vi "labview与三菱PLC通讯(main).vi"(0 "读取=0写入=1":i16, 1 "变量类型":u32(ring) items=["X", "Y", "M", "D"], 2 "PLC地址":string, 3 "PLC数据":string, 4 "16位/32位":u32(ring) items=["16bit", "32bit"], 6 "端口选择":refnum<visa-resource-name>, 8 "波特率":u32(ring) items=["9600"=9600, "19200"=19200, "115200"=115200], 10 "校检":u32(ring) items=["无", "偶", "奇"], 12 "数据位":u32(ring) items=["7"=7, "8"=8]) -> (14 "读取数据输出":u32, 15 "读取成功":bool, 17 "写入成功":bool)   [LabVIEW 2015, in "PLC.lvlib"]
uses:
  PLC.lvlib
panel:
  out "写入PLC变量命令":string
  out "十六进制整型字符串 2":string
  out "十六进制整型字符串":string
  out "长度":i32
  out "数据":string
  out "数字 2":u32
  out "地址偏移量":string="240"
  out "读取PLC变量命令":string
  out "读取为0写入为1":string="1"
  out "校验码2":string
  out "校验码1":string
  out "数字":u16
  out "长度（剩余）":i32=2
  out "变量地址":string
  out "读取返回数据":string
  # "X000-X577"
  # "Y000-Y577"
  # "M0000-M7999"
  # "D0000-D7999"
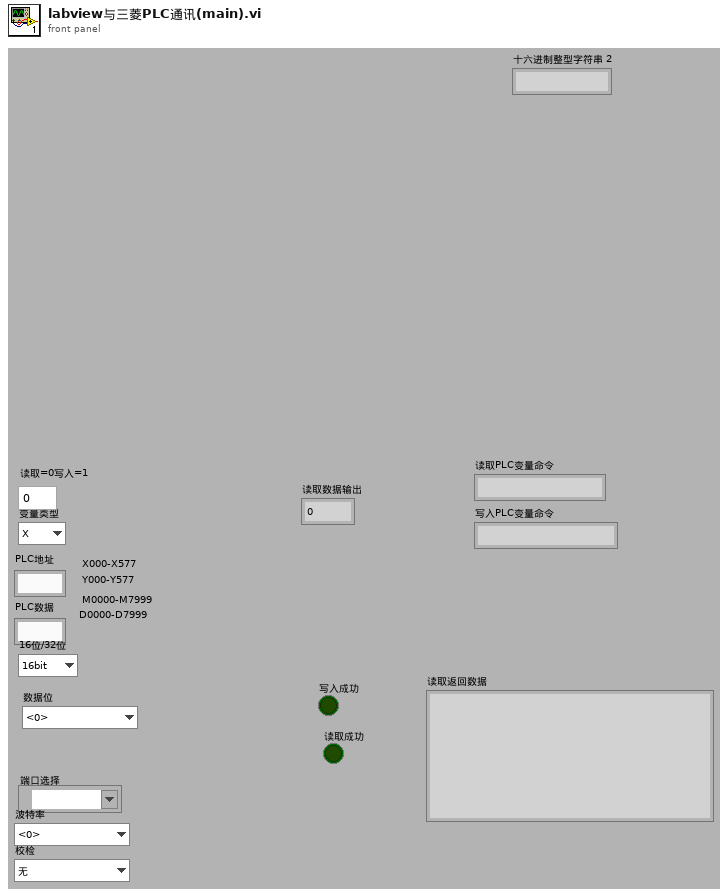
[diagram p1: front panel]
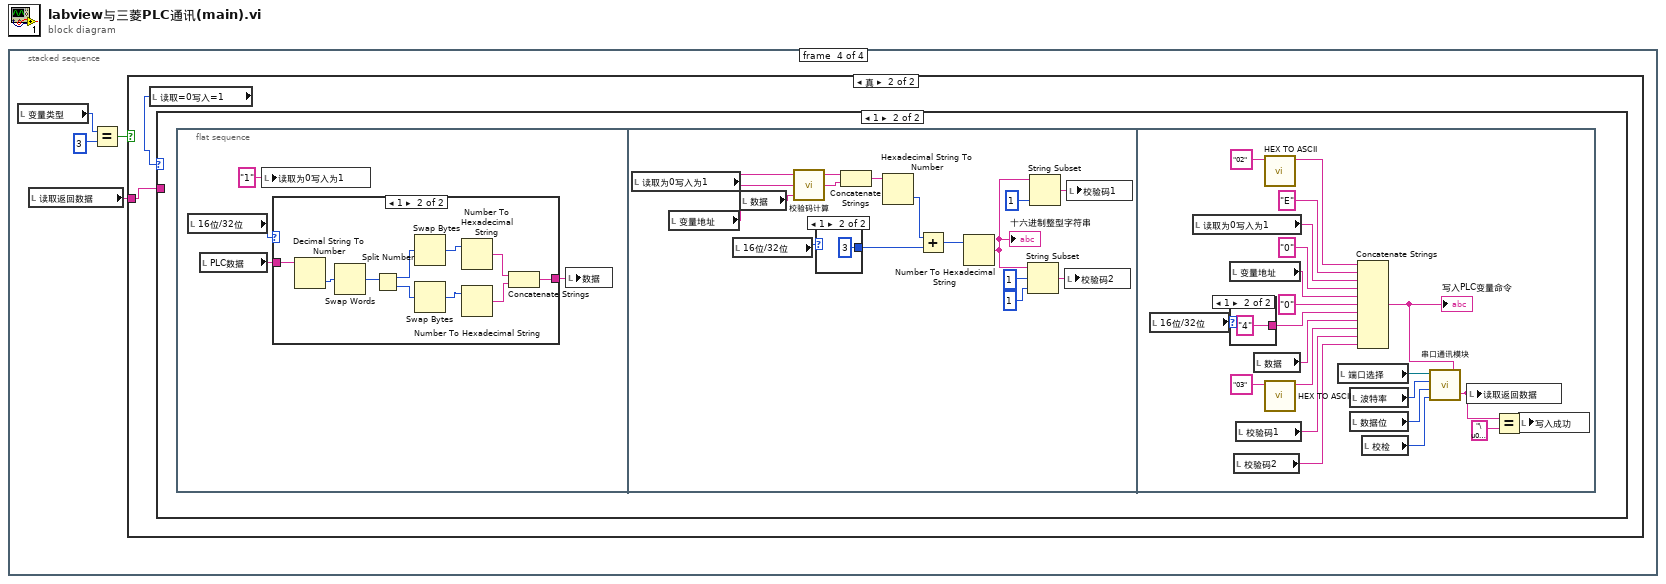
[diagram p0: block diagram]
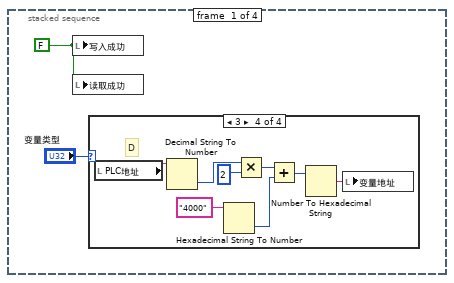
[diagram p2: hidden frame]
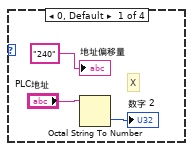
[diagram p3: hidden frame]
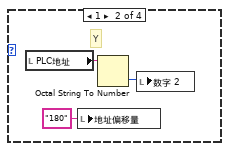
[diagram p4: hidden frame]
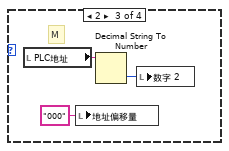
[diagram p5: hidden frame]
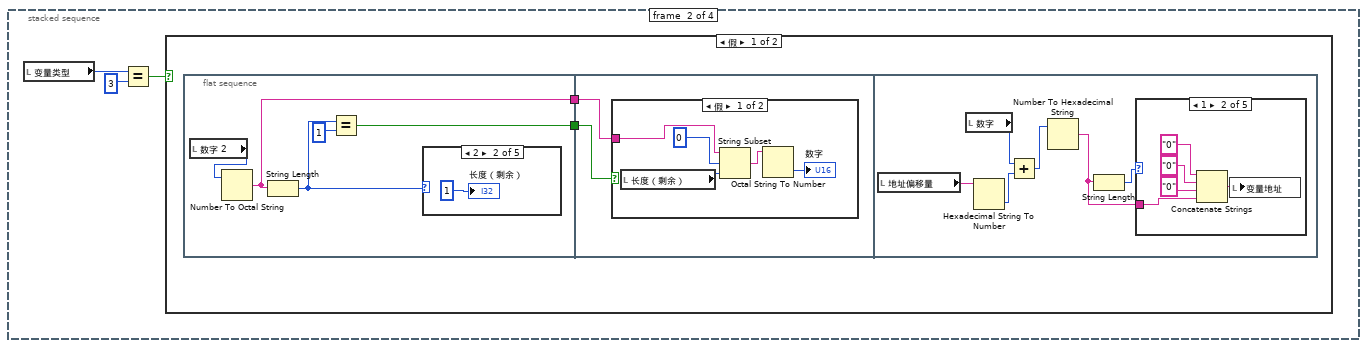
[diagram p6: hidden frame]
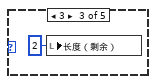
[diagram p8: hidden frame]
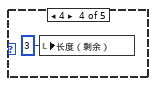
[diagram p9: hidden frame]
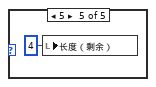
[diagram p10: hidden frame]
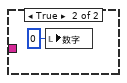
[diagram p11: hidden frame]
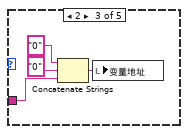
[diagram p13: hidden frame]
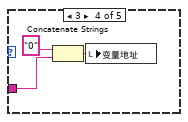
[diagram p14: hidden frame]
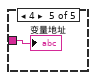
[diagram p15: hidden frame]
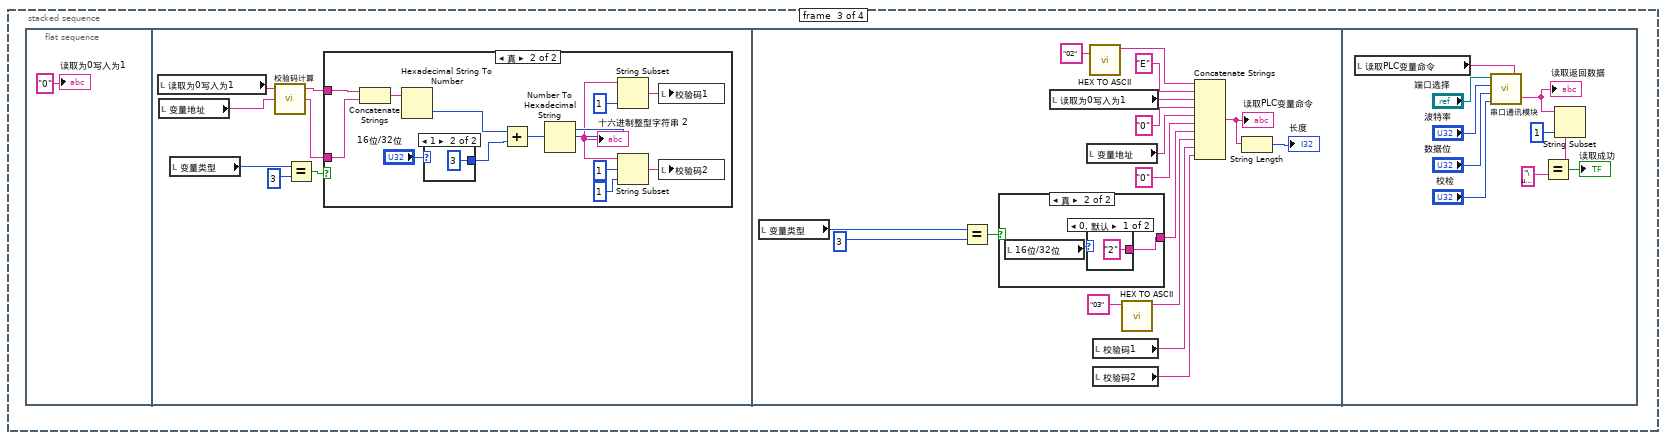
[diagram p17: hidden frame]
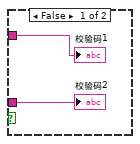
[diagram p18: hidden frame]
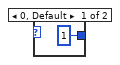
[diagram p19: hidden frame]
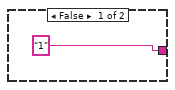
[diagram p20: hidden frame]
diagram:
  n1 = stacked-sequence {
    frame #0 {
      w1 = FALSE ("发送成功")
      n2 = local write "写入成功"(w1) -> ()
      n3 = local write "读取成功"(w1) -> ()
      n4 = case shown="3" "变量类型" {
        frame 0, Default {
          # "X"
          n5 = Octal String To Number(4:"PLC地址") -> (0:→"数字 2":u32)  [unwired: 3 out]
          "地址偏移量" <- "240" ("字符串")
        }
        frame 1 {
          # "Y"
          n6 = local read "PLC地址"() -> (w8:string)
          n7 = local write "地址偏移量"("180" ("字符串")) -> ()
          n8 = Octal String To Number(4:w8) -> (0:w6:u32)  [unwired: 3 out]
          n9 = local write "数字 2"(w6) -> ()
        }
        frame 2 {
          # "M"
          n10 = local read "PLC地址"() -> (w11:string)
          n11 = local write "地址偏移量"("000" ("字符串")) -> ()
          n12 = Decimal String To Number(string=w11) -> (number=w9:i32)  [unwired: 3 out]
          n13 = local write "数字 2"(w9) -> ()
        }
        frame 3 {
          # "D"
          n14 = local read "PLC地址"() -> (w19:string)
          n15 = Decimal String To Number(string=w19) -> (number=w18:i32)  [unwired: 3 out]
          n16 = Hexadecimal String To Number(string="4000" ("PLC地址")) -> (number=w14:u32)  [unwired: 3 out]
          n17 = Multiply(x=w18, y=2) -> (x*y=w15:i32)
          n18 = Add(x=w15, y=w14) -> (x+y=w13:u32)
          n19 = Number To Hexadecimal String(2:w13) -> (0:w12:string)  [unwired: 1 out]
          n20 = local write "变量地址"(w12) -> ()
        }
      }
    }
    frame #1 {
      n21 = local read "变量类型"() -> (w22:u32)
      n22 = Equal?(x=w22, y=u32 3) -> (x = y?=w20:bool)
      n23 = case shown="假" w20 {
        frame False {
          n24 = flat-sequence {
            tunnel: [w28] -> w24
            tunnel: [w27] -> w23
            tunnel: w24 -> [w34]
            tunnel: w23 -> [w35]
            frame #0 {
              n25 = local read "数字 2"() -> (w25:u32)
              n26 = Number To Octal String(2:w25) -> (0:w28:string)  [unwired: 1 out]
              n27 = String Length(string=w28) -> (length=w26:i32)
              n28 = Equal?(x=w26, y=1) -> (x = y?=w27:bool)
              n29 = case shown="2" w26 {
                frame 1, Default {
                }
                frame 2 {
                  "长度（剩余）" <- 1 ("长度（剩余）")
                }
                frame 3 {
                  n30 = local write "长度（剩余）"(2 ("长度（剩余）")) -> ()
                }
                frame 4 {
                  n31 = local write "长度（剩余）"(3 ("长度（剩余）")) -> ()
                }
                frame 5 {
                  n32 = local write "长度（剩余）"(4 ("长度（剩余）")) -> ()
                }
              }
            }
            frame #1 {
              n33 = case shown="假" w35 {
                tunnel: w34 -> [w36 _]
                frame False {
                  n34 = local read "长度（剩余）"() -> (w38:i32)
                  n35 = String Subset(string=w36, offset (0)=0 ("偏移量(0)"), length (rest)=w38) -> (substring=w39:string)
                  n36 = Octal String To Number(4:w39) -> (0:→"数字":u32)  [unwired: 3 out]
                }
                frame True {
                  n37 = local write "数字"(0 ("长度（剩余）")) -> ()
                }
              }
            }
            frame #2 {
              n38 = local read "地址偏移量"() -> (w44:string)
              n39 = local read "数字"() -> (w45:u16)
              n40 = Hexadecimal String To Number(string=w44) -> (number=w47:u32)  [unwired: 3 out]
              n41 = Add(x=w45, y=w47) -> (x+y=w46:u32)
              n42 = Number To Hexadecimal String(2:w46) -> (0:w43:string)  [unwired: 1 out]
              n43 = String Length(string=w43) -> (length=w42:i32)
              n44 = case shown="1" w42 {
                tunnel: w43 -> [_ w48 w53 w57 w60]
                frame 0, Default {
                }
                frame 1 {
                  n45 = Concatenate Strings("0" ("字符串"), "0" ("字符串"), "0" ("字符串"), w48) -> (w49:string)
                  n46 = local write "变量地址"(w49) -> ()
                }
                frame 2 {
                  n47 = Concatenate Strings("0" ("字符串"), "0" ("字符串"), w53) -> (w54:string)
                  n48 = local write "变量地址"(w54) -> ()
                }
                frame 3 {
                  n49 = Concatenate Strings("0" ("字符串"), w57) -> (w58:string)
                  n50 = local write "变量地址"(w58) -> ()
                }
                frame 4 {
                  "变量地址" <- w60
                }
              }
            }
          }
        }
        frame True {
        }
      }
    }
    frame #2 {
      n51 = flat-sequence {
        frame #0 {
          "读取为0写入为1" <- "0" ("字符串")
        }
        frame #1 {
          n52 = local read "读取为0写入为1"() -> (w67:string)
          n53 = local read "变量地址"() -> (w68:string)
          n54 = local read "变量类型"() -> (w64:u32)
          n55 = call "校验码计算.vi"("变量地址"=w68, "读取为0写入为1"=w67) -> ("校验码2"=w62:string, "校验码1"=w63:string)  [unwired: 1 in, 1 out]
          n56 = Equal?(x=w64, y=u32 3) -> (x = y?=w66:bool)
          n57 = case shown="真" w66 {
            tunnel: w62 -> [w70 w75]
            tunnel: w63 -> [w69 w76]
            frame False {
              "校验码1" <- w69
              "校验码2" <- w70
            }
            frame True {
              n58 = Concatenate Strings(w76, w75) -> (w73:string)
              n59 = Hexadecimal String To Number(string=w73) -> (number=w71:u32)  [unwired: 3 out]
              n60 = case shown="1" "16位/32位" {
                tunnel: [u32 1 ("y") u32 3 ("y")] -> w72
                frame 0, Default {
                }
                frame 1 {
                }
              }
              n61 = Add(x=w71, y=w72) -> (x+y=w83:u32)
              n62 = Number To Hexadecimal String(2:w83) -> (0:w82:string)  [unwired: 1 out]
              "十六进制整型字符串 2" <- w82
              n63 = String Subset(string=w82, length (rest)=1 ("长度（剩余）")) -> (substring=w77:string)  [unwired: 1 out]
              n64 = String Subset(string=w82, offset (0)=1 ("偏移量(0)"), length (rest)=1 ("长度（剩余）")) -> (substring=w78:string)
              n65 = local write "校验码1"(w77) -> ()
              n66 = local write "校验码2"(w78) -> ()
            }
          }
        }
        frame #2 {
          n67 = local read "变量类型"() -> (w89:u32)
          n68 = Equal?(x=w89, y=u32 3) -> (x = y?=w87:bool)
          n69 = case shown="真" w87 {
            tunnel: ["1" ("字符串") w104] -> w86
            frame False {
            }
            frame True {
              n70 = local read "16位/32位"() -> (w105:u32)
              n71 = case shown="0, 默认" w105 {
                tunnel: ["2" ("y") "4" ("y")] -> w104
                frame 0, Default {
                }
                frame 1 {
                }
              }
            }
          }
          n72 = local read "读取为0写入为1"() -> (w102:string)
          n73 = local read "变量地址"() -> (w99:string)
          n74 = call "HEX TO ASCII.vi"("HEX"="02") -> ("ASCII"=w97:string)  [unwired: 10 out]
          n75 = local read "校验码1"() -> (w100:string)
          n76 = local read "校验码2"() -> (w101:string)
          n77 = call "HEX TO ASCII.vi"("HEX"="03") -> ("ASCII"=w98:string)  [unwired: 10 out]
          n78 = Concatenate Strings(w97, "E" ("字符串"), w102, "0" ("字符串"), w99, "0" ("字符串"), w86, w98, w100, w101) -> (w90:string)
          "读取PLC变量命令" <- w90
          n79 = String Length(string=w90) -> (length=→"长度":i32)
        }
        frame #3 {
          n80 = local read "读取PLC变量命令"() -> (w111:string)
          n81 = call "串口通讯模块.vi"("发送区"=w111, "校检"="校检", "数据位"="数据位", "波特率"="波特率", "VISA resource name"="端口选择") -> ("接收区"=w117:string)  [unwired: 2 out]
          "读取返回数据" <- w117
          n82 = String Subset(string=w117, length (rest)=1 ("长度（剩余）")) -> (substring=w115:string)  [unwired: 1 out]
          n83 = Equal?(x=w115, y="\u0002" ("字符串")) -> (x = y?=→"读取成功":bool)
        }
      }
    }
    frame #3 {
      n84 = local read "变量类型"() -> (w121:u32)
      n85 = local read "读取返回数据"() -> (w118:string)
      n86 = Equal?(x=w121, y=u32 3) -> (x = y?=w119:bool)
      n87 = case shown="真" w119 {
        tunnel: w118 -> [w122 w233]
        frame False {
          n88 = case shown="1" "读取=0写入=1" {
            tunnel: w122 -> [w124 w159]
            frame 0, Default {
              n89 = local read "PLC地址"() -> (w126:string)
              n90 = String Length(string=w126) -> (length=w127:i32)
              n91 = local write "读取为0写入为1"("0" ("读取为0写入为1")) -> ()
              n92 = case shown="1" w127 {
                tunnel: w126 -> [_ w150 w153 w156]
                tunnel: [_ w148 w151 w155] -> w125
                frame 0, Default {
                }
                frame 1 {
                  n93 = String Subset(string=w150, length (rest)=1 ("长度（剩余）")) -> (substring=w148:string)  [unwired: 1 out]
                }
                frame 2 {
                  n94 = String Subset(string=w153, offset (0)=1 ("偏移量(0)"), length (rest)=1 ("长度（剩余）")) -> (substring=w151:string)
                }
                frame 3 {
                  n95 = String Subset(string=w156, offset (0)=2 ("偏移量(0)"), length (rest)=1 ("长度（剩余）")) -> (substring=w155:string)
                }
              }
              n96 = String Subset(string=w124, offset (0)=1 ("偏移量(0)"), length (rest)=2 ("长度（剩余）")) -> (substring=w129:string)
              n97 = Hexadecimal String To Number(string=w129) -> (number=w128:u32)  [unwired: 3 out]
              n98 = case shown="\"2\"" w125 {
                tunnel: [_ 0 ("长度（剩余）") 1 ("长度（剩余）") 2 ("长度（剩余）") 3 ("长度（剩余）") 4 ("长度（剩余）") 5 ("长度（剩余）") 6 ("长度（剩余）") 7 ("长度（剩余）")] -> w133
                frame "假", Default {
                }
                frame "0" {
                }
                frame "1" {
                }
                frame "2" {
                }
                frame "3" {
                }
                frame "4" {
                }
                frame "5" {
                }
                frame "6" {
                }
                frame "7" {
                }
              }
              n99 = Number To Boolean Array(number=w128) -> (Boolean array=w134:bool[])
              n100 = Index Array(array=w134, index=w133) -> (element=w135:bool)
              n101 = Equal?(x=w135, y=TRUE) -> (x = y?=w137:bool)
              n102 = case shown="假" w137 {
                frame False {
                  n103 = local write "读取数据输出"(u32 0 ("读取数据输出")) -> ()
                }
                frame True {
                  n104 = local write "读取数据输出"(u32 1 ("读取数据输出")) -> ()
                }
              }
            }
            frame 1 {
              n105 = flat-sequence {
                tunnel: w159 -> [w160]
                frame #0 {
                  n106 = local read "PLC地址"() -> (w167:string)
                  n107 = local read "变量类型"() -> (w164:u32)
                  n108 = String Length(string=w167) -> (length=w168:i32)
                  n109 = Equal?(x=w164, y=u32 3) -> (x = y?=w163:bool)
                  n110 = case shown="1" w168 {
                    tunnel: w167 -> [_ w197 w200 w203]
                    tunnel: [_ w195 w198 w202] -> w166
                    frame 0, Default {
                    }
                    frame 1 {
                      n111 = String Subset(string=w197, length (rest)=1 ("长度（剩余）")) -> (substring=w195:string)  [unwired: 1 out]
                    }
                    frame 2 {
                      n112 = String Subset(string=w200, offset (0)=1 ("偏移量(0)"), length (rest)=1 ("长度（剩余）")) -> (substring=w198:string)
                    }
                    frame 3 {
                      n113 = String Subset(string=w203, offset (0)=2 ("偏移量(0)"), length (rest)=1 ("长度（剩余）")) -> (substring=w202:string)
                    }
                  }
                  n114 = case shown="假" w163 {
                    tunnel: [w183 _] -> w161
                    frame False {
                      n115 = case shown="\"1\"" "PLC数据" {
                        tunnel: [_ FALSE ("新元素/子数组") TRUE ("新元素/子数组")] -> w183
                        frame "假", Default {
                        }
                        frame "0" {
                        }
                        frame "1" {
                        }
                      }
                    }
                    frame True {
                    }
                  }
                  n116 = String Subset(string=w160, offset (0)=1 ("偏移量(0)"), length (rest)=2 ("长度（剩余）")) -> (substring=w173:string)
                  n117 = Hexadecimal String To Number(string=w173) -> (number=w172:u32)  [unwired: 3 out]
                  n118 = case shown="\"6\"" w166 {
                    tunnel: [_ 0 ("长度（剩余）") 1 ("长度（剩余）") 2 ("长度（剩余）") 3 ("长度（剩余）") 4 ("长度（剩余）") 5 ("长度（剩余）") 6 ("长度（剩余）") 7 ("长度（剩余）")] -> w165
                    frame "假", Default {
                    }
                    frame "0" {
                    }
                    frame "1" {
                    }
                    frame "2" {
                    }
                    frame "3" {
                    }
                    frame "4" {
                    }
                    frame "5" {
                    }
                    frame "6" {
                    }
                    frame "7" {
                    }
                  }
                  n119 = Number To Boolean Array(number=w172) -> (Boolean array=w171:bool[])
                  n120 = Replace Array Subset(array=w171, new element=w161, index=w165) -> (w170:bool[])
                  n121 = Boolean Array To Number(Boolean array=w170) -> (number=w169:u32)
                  n122 = local write "读取为0写入为1"("1" ("读取为0写入为1")) -> ()
                  n123 = Number To Hexadecimal String(2:w169) -> (0:w178:string)  [unwired: 1 out]
                  n124 = String Length(string=w178) -> (length=w177:i32)
                  n125 = case shown="1" w177 {
                    tunnel: w178 -> [_ w180 w182]
                    frame 0, Default {
                    }
                    frame 1 {
                      n126 = Concatenate Strings("0" ("字符串"), w180) -> (→"数据":string)
                    }
                    frame 2 {
                      n127 = local write "数据"(w182) -> ()
                    }
                  }
                }
                frame #1 {
                  n128 = local read "读取为0写入为1"() -> (w208:string)
                  n129 = local read "变量地址"() -> (w209:string)
                  n130 = local read "数据"() -> (w210:string)
                  n131 = call "校验码计算.vi"("变量数据"=w210, "变量地址"=w209, "读取为0写入为1"=w208) -> ("校验码2"=w206:string, "校验码1"=w207:string)  [unwired: 1 out]
                  n132 = local write "校验码1"(w207) -> ()
                  n133 = local write "校验码2"(w206) -> ()
                }
                frame #2 {
                  n134 = local read "读取为0写入为1"() -> (w231:string)
                  n135 = local read "变量地址"() -> (w227:string)
                  n136 = local read "校验码1"() -> (w229:string)
                  n137 = local read "校验码2"() -> (w230:string)
                  n138 = local read "数据"() -> (w214:string)
                  n139 = call "HEX TO ASCII.vi"("HEX"="02") -> ("ASCII"=w225:string)  [unwired: 10 out]
                  n140 = call "HEX TO ASCII.vi"("HEX"="03") -> ("ASCII"=w226:string)  [unwired: 10 out]
                  n141 = local read "端口选择"() -> (w218:refnum<visa-resource-name>)
                  n142 = Concatenate Strings(w225, "E" ("字符串"), w231, "0" ("字符串"), w227, "0" ("字符串"), "1" ("字符串"), w214, w226, w229, w230) -> (w219:string)
                  n143 = local read "波特率"() -> (w217:u32)
                  n144 = local read "数据位"() -> (w216:u32)
                  n145 = local read "校检"() -> (w215:u32)
                  n146 = call "串口通讯模块.vi"("发送区"=w219, "校检"=w215, "数据位"=w216, "波特率"=w217, "VISA resource name"=w218) -> ("接收区"=w211:string)  [unwired: 2 out]
                  n147 = local write "读取返回数据"(w211) -> ()
                  n148 = Equal?(x=w211, y="\u0006" ("接收区 2")) -> (x = y?=→"写入成功":bool)
                }
              }
            }
          }
        }
        frame True {
          n149 = local read "读取=0写入=1"() -> (w232:i16)
          n150 = case shown="1" w232 {
            tunnel: w233 -> [w234 _]
            frame 0, Default {
              n151 = String Length(string=w234) -> (length=w235:i32)
              n152 = case shown="8, 默认" w235 {
                tunnel: w234 -> [w236 w254]
                frame 8, Default {
                  n153 = String Subset(string=w236, offset (0)=1 ("偏移量(0)"), length (rest)=4 ("长度（剩余）")) -> (substring=w241:string)
                  n154 = Hexadecimal String To Number(string=w241) -> (number=w237:u32)  [unwired: 3 out]
                  n155 = Swap Bytes(anything=w237) -> (byte swapped=→"读取数据输出":u32)
                }
                frame 12 {
                  n156 = String Subset(string=w254, offset (0)=1 ("偏移量(0)"), length (rest)=8 ("长度（剩余）")) -> (substring=w257:string)
                  n157 = Hexadecimal String To Number(string=w257) -> (number=w251:u32)  [unwired: 3 out]
                  n158 = Swap Words(1:w251) -> (0:w253:u32)
                  n159 = Split Number(x=w253) -> (hi(x)=w248:u16, lo(x)=w252:u16)
                  n160 = Swap Bytes(anything=w252) -> (byte swapped=w247:u16)
                  n161 = Swap Bytes(anything=w248) -> (byte swapped=w246:u16)
                  n162 = Number To Hexadecimal String(2:w246) -> (0:w244:string)  [unwired: 1 out]
                  n163 = Number To Hexadecimal String(2:w247) -> (0:w249:string)  [unwired: 1 out]
                  n164 = String Length(string=w249) -> (length=w250:i32)
                  n165 = case shown="0, 默认" w250 {
                    tunnel: ["0000" w259 w262 w266 w268] -> w245
                    tunnel: w249 -> [_ w261 w263 w265 w268]
                    frame 0, Default {
                    }
                    frame 1 {
                      n166 = Concatenate Strings("000" ("字符串"), w261) -> (w259:string)
                    }
                    frame 2 {
                      n167 = Concatenate Strings("00" ("字符串"), w263) -> (w262:string)
                    }
                    frame 3 {
                      n168 = Concatenate Strings("0" ("字符串"), w265) -> (w266:string)
                    }
                    frame 4 {
                    }
                  }
                  n169 = Concatenate Strings(w244, w245) -> (w243:string)
                  n170 = Hexadecimal String To Number(string=w243) -> (number=w242:u32)  [unwired: 3 out]
                  n171 = local write "读取数据输出"(w242) -> ()
                }
              }
            }
            frame 1 {
              n172 = flat-sequence {
                frame #0 {
                  n173 = local read "16位/32位"() -> (w270:u32)
                  n174 = local read "PLC数据"() -> (w272:string)
                  n175 = local write "读取为0写入为1"("1" ("读取为0写入为1")) -> ()
                  n176 = case shown="1" w270 {
                    tunnel: w272 -> [w276 w285]
                    tunnel: [w274 w286] -> w269
                    frame 0, Default {
                      n177 = Decimal String To Number(string=w276) -> (number=w278:i32)  [unwired: 3 out]
                      n178 = Swap Bytes(anything=w278) -> (byte swapped=w277:i32)
                      n179 = Number To Hexadecimal String(2:w277) -> (0:w275:string)  [unwired: 1 out]
                      n180 = String Subset(string=w275, length (rest)=4 ("长度（剩余）")) -> (substring=w274:string)  [unwired: 1 out]
                    }
                    frame 1 {
                      n181 = Decimal String To Number(string=w285) -> (number=w284:i32)  [unwired: 3 out]
                      n182 = Swap Words(1:w284) -> (0:w283:i32)
                      n183 = Split Number(x=w283) -> (hi(x)=w288:u16, lo(x)=w287:u16)
                      n184 = Swap Bytes(anything=w288) -> (byte swapped=w281:u16)
                      n185 = Swap Bytes(anything=w287) -> (byte swapped=w282:u16)
                      n186 = Number To Hexadecimal String(2:w281) -> (0:w280:string)  [unwired: 1 out]
                      n187 = Number To Hexadecimal String(2:w282) -> (0:w279:string)  [unwired: 1 out]
                      n188 = Concatenate Strings(w280, w279) -> (w286:string)
                    }
                  }
                  n189 = local write "数据"(w269) -> ()
                }
                frame #1 {
                  n190 = local read "读取为0写入为1"() -> (w303:string)
                  n191 = local read "变量地址"() -> (w304:string)
                  n192 = local read "16位/32位"() -> (w290:u32)
                  n193 = local read "数据"() -> (w302:string)
                  n194 = call "校验码计算.vi"("变量数据"=w302, "变量地址"=w304, "读取为0写入为1"=w303) -> ("校验码2"=w300:string, "校验码1"=w301:string)  [unwired: 1 out]
                  n195 = case shown="1" w290 {
                    tunnel: [u32 1 ("y") u32 3 ("y")] -> w289
                    frame 0, Default {
                    }
                    frame 1 {
                    }
                  }
                  n196 = Concatenate Strings(w301, w300) -> (w299:string)
                  n197 = Hexadecimal String To Number(string=w299) -> (number=w298:u32)  [unwired: 3 out]
                  n198 = Add(x=w298, y=w289) -> (x+y=w297:u32)
                  n199 = Number To Hexadecimal String(2:w297) -> (0:w296:string)  [unwired: 1 out]
                  "十六进制整型字符串" <- w296
                  n200 = String Subset(string=w296, offset (0)=1 ("偏移量(0)"), length (rest)=1 ("长度（剩余）")) -> (substring=w292:string)
                  n201 = String Subset(string=w296, length (rest)=1 ("长度（剩余）")) -> (substring=w291:string)  [unwired: 1 out]
                  n202 = local write "校验码2"(w292) -> ()
                  n203 = local write "校验码1"(w291) -> ()
                }
                frame #2 {
                  n204 = local read "16位/32位"() -> (w308:u32)
                  n205 = local read "读取为0写入为1"() -> (w327:string)
                  n206 = local read "变量地址"() -> (w324:string)
                  n207 = case shown="1" w308 {
                    tunnel: ["2" ("字符串") "4" ("字符串")] -> w307
                    frame 0, Default {
                    }
                    frame 1 {
                    }
                  }
                  n208 = local read "校验码2"() -> (w326:string)
                  n209 = local read "校验码1"() -> (w325:string)
                  n210 = local read "数据"() -> (w311:string)
                  n211 = call "HEX TO ASCII.vi"("HEX"="02") -> ("ASCII"=w322:string)  [unwired: 10 out]
                  n212 = call "HEX TO ASCII.vi"("HEX"="03") -> ("ASCII"=w323:string)  [unwired: 10 out]
                  n213 = local read "端口选择"() -> (w315:refnum<visa-resource-name>)
                  n214 = local read "波特率"() -> (w314:u32)
                  n215 = local read "数据位"() -> (w313:u32)
                  n216 = Concatenate Strings(w322, "E" ("字符串"), w327, "0" ("字符串"), w324, "0" ("字符串"), w307, w311, w323, w325, w326) -> (w316:string)
                  "写入PLC变量命令" <- w316
                  n217 = local read "校检"() -> (w312:u32)
                  n218 = call "串口通讯模块.vi"("发送区"=w316, "校检"=w312, "数据位"=w313, "波特率"=w314, "VISA resource name"=w315) -> ("接收区"=w309:string)  [unwired: 2 out]
                  n219 = local write "读取返回数据"(w309) -> ()
                  n220 = Equal?(x=w309, y="\u0006" ("接收区 2")) -> (x = y?=w328:bool)
                  n221 = local write "写入成功"(w328) -> ()
                }
              }
            }
          }
        }
      }
    }
  }
